vi "Status Questionable Enable.vi"(0 "VISA resource name":refnum<visa-resource-name>, 7 "SQER (All F:Disable)":bool[](array[boolean])=[FALSE, FALSE, FALSE, FALSE, FALSE], 11 "error in (no error)":errorcluster) -> (4 "VISA resource name out":refnum<visa-resource-name>, 15 "error out":errorcluster)   [LabVIEW 2015, in "Chroma ATE 6310.lvlib"]
doc: "Mask for selecting which bits on the Event register are allowed to be summed into the QUES bit of the Status Byte register."
uses:
  <instrlib>/Chroma ATE 6310/Chroma ATE 6310.lvlib
panel:
  # "CE                VE                 PE                 RV                TE"
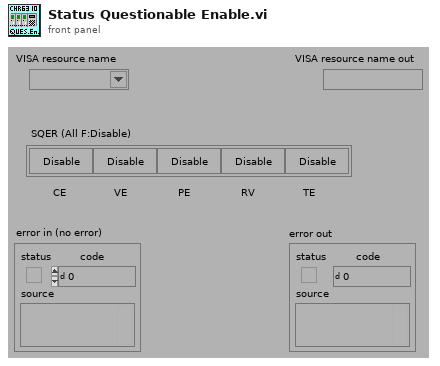
[diagram p1: front panel]
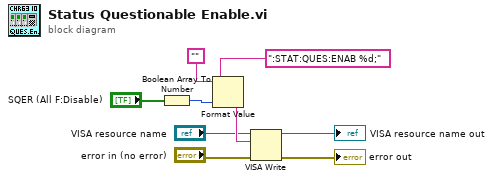
[diagram p0: block diagram]
diagram:
  n1 = Boolean Array To Number(Boolean array="SQER (All F:Disable)") -> (number=w6:u32)
  n2 = Format Value(string ("")="", format string=":STAT:QUES:ENAB %d;", value (0)=w6) -> (output string=w7:string)
  n3 = VISA Write(VISA resource name="VISA resource name", write buffer=w7, error in (no error)="error in (no error)") -> (VISA resource name out=→"VISA resource name out":refnum<visa-resource-name>, error out=→"error out":errorcluster)  [unwired: 1 out]
